vi "read_table_key_string.vi"(7 "table":string, 8 "error in (no error)":errorcluster, 9 "default (\"\")":string, 10 "key":string, 11 "toml in":refnum<class "toml.lvclass">) -> (0 "error out":errorcluster, 1 "value":string, 3 "toml out":refnum<class "toml.lvclass">)   [LabVIEW 2020, in "toml.lvclass"]
uses:
  toml.lvclass
  toml.lvclass/toml.ctl
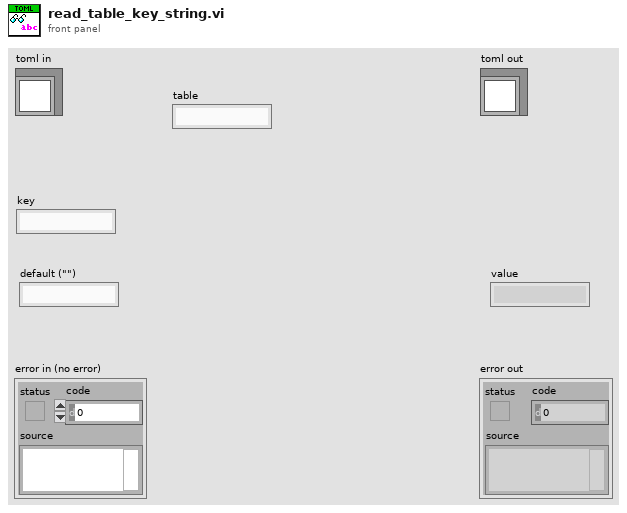
[diagram p1: front panel]
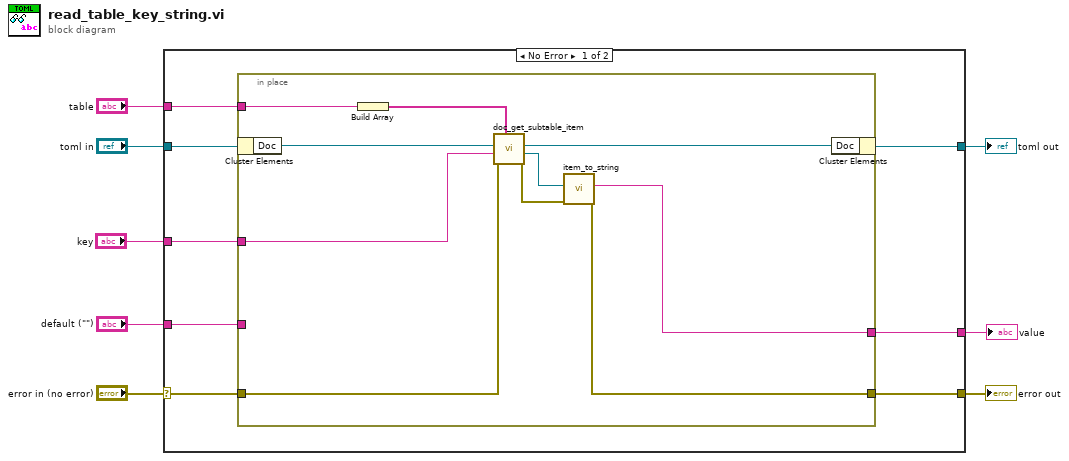
[diagram p0: block diagram]
diagram:
  n1 = case shown="No Error" "error in (no error)" {
    selector: "error in (no error)" -> [w10 w28]
    tunnel: [w11 w28] -> w7
    tunnel: [w15 w27] -> w5
    tunnel: "toml in" -> [w16 w27]
    tunnel: "table" -> [w14 _]
    tunnel: "key" -> [w13 _]
    tunnel: "default (\"\")" -> [w12 _]
    tunnel: [w9 _] -> w1
    frame No Error {
      n2 = in-place {
        in-place-border: w14 -> [w24]
        in-place-border: w13 -> [w21]
        in-place-border: w12 -> [_]
        in-place-border: [w17] -> w11
        in-place-border: w10 -> [w22]
        in-place-border: [w19] -> w9
        n3 = in-place-cluster #1(w16) -> ("Doc"=w26:refnum<class "Doc.lvclass">)
        n4 = Build Array(w24) -> (w23:string[])
        n5 = call "doc_get_subtable_item.vi"("subtables"=w23, "error in (no error)"=w22, "key"=w21, "Doc in"=w26) -> ("error out"=w18:errorcluster, "item (value)"=w20:refnum<class "Item.lvclass">, "Doc out"=w25:refnum<class "Doc.lvclass">)  [unwired: 5 in]
        n6 = call "item_to_string.vi"("error in (no error)"=w18, "Item in"=w20) -> ("error out"=w17:errorcluster, "string_value"=w19:string)  [unwired: 8 in]
        n7 = in-place-cluster #1("Doc"=w25) -> (w15:refnum<class "toml.lvclass">)
      }
    }
    frame Error {
    }
  }
  "error out" <- w7
  "toml out" <- w5
  "value" <- w1
